vi "Process Data PID 0 Ative_vel.vi"(0 "A Pos":i32, 7 "Target Pos":i32, 9 "Profile Vel":i32, 11 "dt IN(s)":dbl, 12 "PID SET":T1) -> (4 "Target velocity":i32, 15 "dt OUT(s)":dbl)   [LabVIEW 2019]
uses:
  <vilib>/addons/control/pid/pid.llb/PID (DBL).vi
  <vilib>/addons/control/pid/NI_PID_pid.lvlib
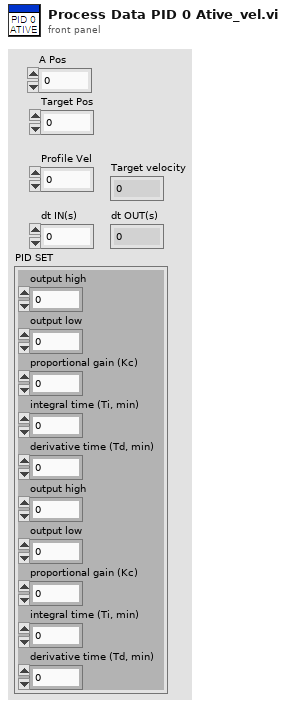
[diagram p1: front panel]
types:
  T1 = cluster{"output high":dbl, "output low":dbl, "proportional gain (Kc)":dbl, "integral time (Ti, min)":dbl, "derivative time (Td, min)":dbl, "output high":dbl, "output low":dbl, "proportional gain (Kc)":dbl, "integral time (Ti, min)":dbl, "derivative time (Td, min)":dbl}
  T2 = cluster{"proportional gain (Kc)":dbl, "integral time (Ti, min)":dbl, "derivative time (Td, min)":dbl}
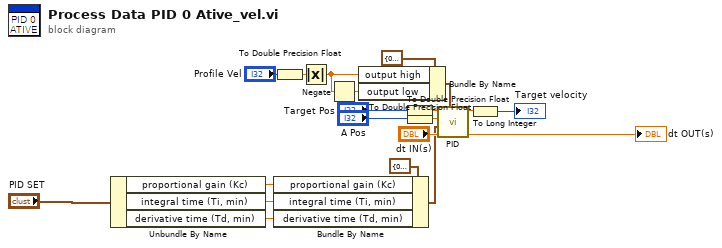
[diagram p0: block diagram]
diagram:
  n1 = Unbundle By Name("PID SET") -> ("proportional gain (Kc)"=w8:dbl, "integral time (Ti, min)"=w6:dbl, "derivative time (Td, min)"=w7:dbl)
  n2 = Bundle By Name(cluster=T2 {"proportional gain (Kc)"=0.0, "integral time (Ti, min)"=0.0, "derivative time (Td, min)"=0.0} ("PID gains"), "proportional gain (Kc)"=w8, "integral time (Ti, min)"=w6, "derivative time (Td, min)"=w7) -> (w15:T2)
  n3 = To Double Precision Float(number="Profile Vel") -> (double precision float=w19:dbl)
  n4 = Absolute Value(x=w19) -> (abs(x)=w18:dbl)
  n5 = Negate(x=w18) -> (-x=w17:dbl)
  n6 = Bundle By Name(cluster=cluster{"output high":dbl, "output low":dbl} {"output high"=0.0, "output low"=0.0} ("output range"), "output high"=w18, "output low"=w17) -> (w10:cluster{"output high":dbl, "output low":dbl})
  n7 = To Double Precision Float(number="Target Pos") -> (double precision float=w11:dbl)
  n8 = To Double Precision Float(number="A Pos") -> (double precision float=w13:dbl)
  n9 = call-poly <vilib>:"PID.vi"("output range"=w10, "dt (s)"="dt IN(s)", "PID gains"=w15, "process variable"=w13, "setpoint"=w11) -> ("dt out (s)"=→"dt OUT(s)":dbl, "output"=w2:dbl)  [unwired: 5 in]
  n10 = To Long Integer(number=w2) -> (32bit integer=→"Target velocity":i32)
